vi "Communication - FTDI Command (eFGV).vi"(7 "Action":T3, 8 "error in":errorcluster, 10 "Fron?":bool, 11 "FDTI CMD":T1) -> (0 "error out":errorcluster, 2 "FDTI ref":refnum<user-event>, 3 "FDTI Out":T1)   [LabVIEW 2019]
uses:
  Controls/eFGV States.ctl
  Controls/FTDI - Communication.ctl
  Controls/UDP - Command.ctl
  <vilib>/event_ctls.llb/usereventprio.ctl
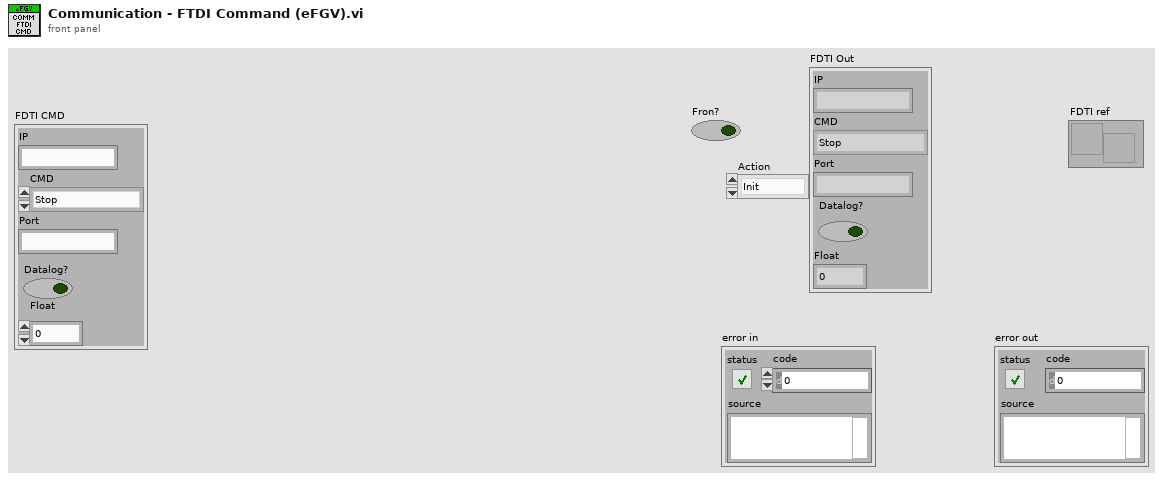
[diagram p1: front panel]
types:
  T1 = typedef "FTDI - Communication.ctl" = cluster{"IP":string, "CMD":T2, "Port":string, "Datalog?":bool, "Float":dbl}
  T2 = typedef "UDP - Command.ctl" = enum16{"Stop", "Jog Up", "Jog Down", "Ramp Up", "Ramp Down", "PID Target", "PID Ramp", "Disp Run", "Read Ch Data", "Zero Channel", "Zero Disp", "Read Sensor", "Write Sensor", "Read ADC", "Write ADC", "Read PID", "Write PID", "Read Test", "Write Test", "Read System", "Write System", "Read Datalog", "Read Datalog Sensor"}
  T3 = typedef "eFGV States.ctl" = enum16{"Init", "Read", "Write", "Exit"}
  T4 = typedef "usereventprio.ctl" = enum32{"high priority", "normal priority"}
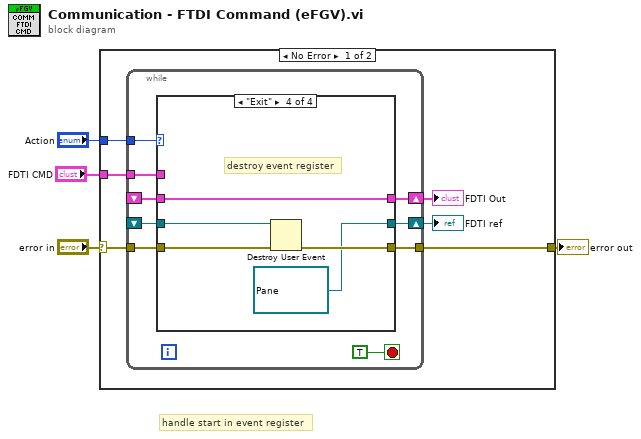
[diagram p0: block diagram]
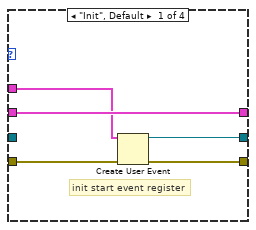
[diagram p2: hidden frame]
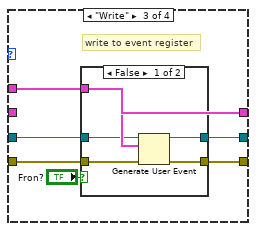
[diagram p4: hidden frame]
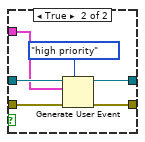
[diagram p5: hidden frame]
diagram:
  # "handle start in event register"
  n1 = case shown="No Error" "error in" {
    selector: "error in" -> [w8 w50]
    tunnel: "Action" -> [w10 _]
    tunnel: "FDTI CMD" -> [w7 _]
    tunnel: [w9 w50] -> w3
    frame No Error {
      n2 = while {
        tunnel: w10 -> [w18]
        tunnel: w8 -> [w16]
        tunnel: [w15] -> w9
        shift-right: [w14] -> w5
        shift-left: _ -> [w17]
        tunnel: w7 -> [w13]
        shift-right: [w12] -> w6
        shift-left: _ -> [w11]
        stop <- TRUE stop-if-true
        n3 = case shown="\"Exit\"" w18 {
          tunnel: w17 -> [w24 w26 _ w46]
          tunnel: w16 -> [w23 w27 w30 w49]
          tunnel: [w22 w27 w33 w48] -> w15
          tunnel: [w24 w26 w32 w46] -> w14
          tunnel: w13 -> [w21 _ w32 _]
          tunnel: w11 -> [_ w25 w31 w47]
          tunnel: [w20 w25 w28 refnum<user-event> refnum ("FDTI CMD")] -> w12
          frame "Init", Default {
            # "init start event register"
            n4 = Create User Event(user event datatype=w21, error in=w23) -> (user event=w20:refnum<user-event>, error out=w22:errorcluster)
          }
          frame "Read" {
            # "read from event register"
          }
          frame "Write" {
            # "write to event register"
            n5 = case shown="False" "Fron?" {
              tunnel: [w38 w43] -> w33
              tunnel: w32 -> [w37 w40]
              tunnel: w31 -> [w36 w42]
              tunnel: w30 -> [w35 w44]
              tunnel: [w34 w41] -> w28
              frame False {
                n6 = Generate User Event(user event=w36, event data cluster=w37, error in=w35) -> (user event out=w34:refnum<user-event>, error out=w38:errorcluster)  [unwired: 1 in]
              }
              frame True {
                n7 = Generate User Event(priority (normal)=usereventprio."high priority", user event=w42, event data cluster=w40, error in=w44) -> (user event out=w41:refnum<user-event>, error out=w43:errorcluster)
              }
            }
          }
          frame "Exit" {
            # "destroy event register"
            n8 = Destroy User Event(user event=w47, error in=w49) -> (error out=w48:errorcluster)
          }
        }
      }
      "FDTI ref" <- w6
      "FDTI Out" <- w5
    }
    frame Error {
    }
  }
  "error out" <- w3
